vi "PC_DynamicCallRTVI.vi"   [LabVIEW 2010]
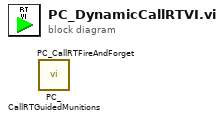
[diagram p0: block diagram]
diagram:
  n1 = call "PC_CallRTGuidedMunitions.vi"() -> ()  [unwired: 10 in, 2 out]
  n2 = call "PC_CallRTFireAndForget.vi"() -> ()  [unwired: 10 in, 2 out]
